vi "Data read test-Crossrulz.vi"() -> ()   [LabVIEW 2020]
uses:
  <vilib>/Instr/_visa.llb/VISA Configure Serial Port (Instr).vi
panel:
  out "Msg ID":string
  out "Header":string
  out "unsigned byte array":u8[](array[numeric])
  in  "Multicolumn Listbox":i32(listbox)
  out "error out":errorcluster
  in  "stop":bool
  in  "VISA resource name":refnum<visa-resource-name>
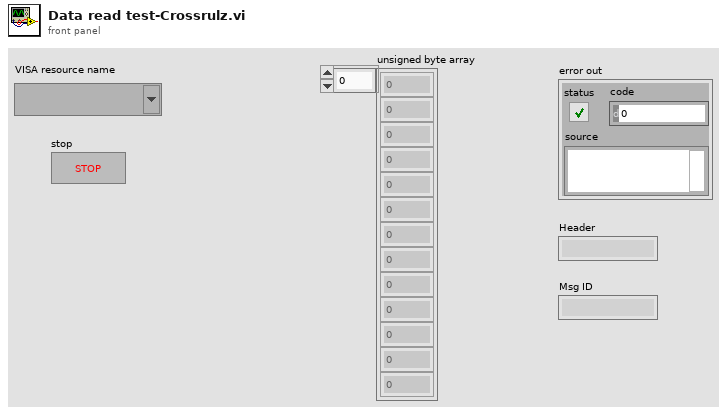
[diagram p1: front panel]
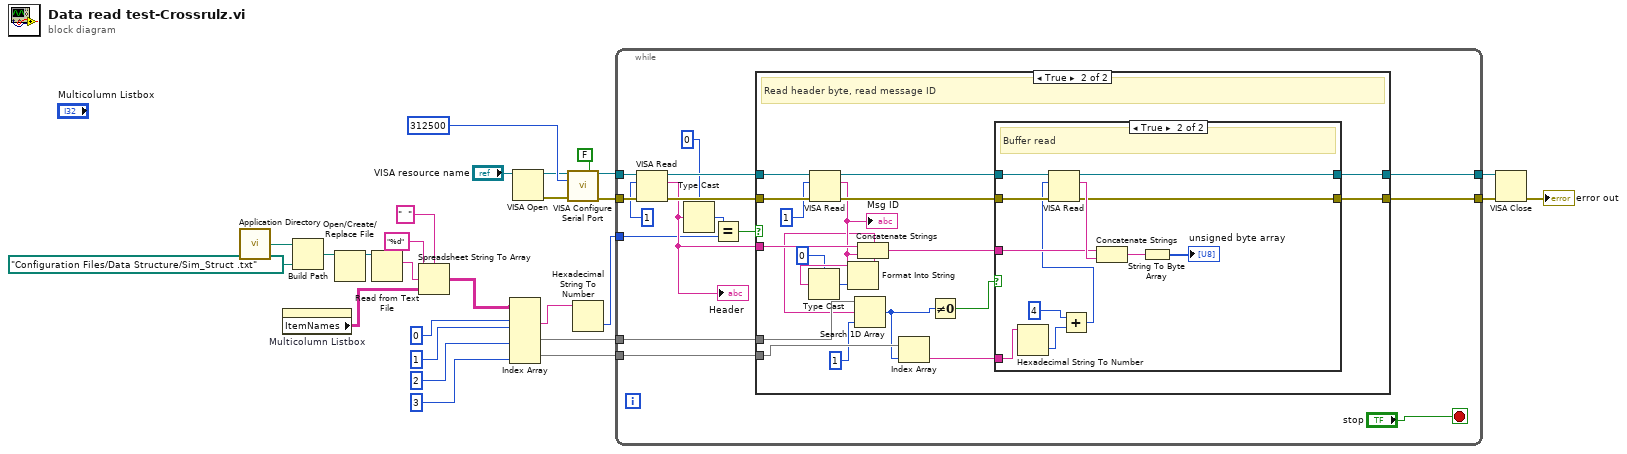
[diagram p0: block diagram]
diagram:
  n1 = call <vilib>:"Application Directory.vi"() -> ("Application Directory"=w16:path)
  n2 = property on="Multicolumn Listbox" class="MCListbox (strict)"() -> ("ItemNames"=w9:string[][])  [unwired: 2 in, 2 out]
  n3 = Build Path(base path=w16, name or relative path=path "Configuration Files/Data Structure/Sim_Struct .txt") -> (appended path=w14:path)
  n4 = Open/Create/Replace File(file path (use dialog)=w14) -> (refnum out=w13:refnum<file>)  [unwired: 5 in, 2 out]
  n5 = Read from Text File(file (use dialog)=w13) -> (text=w12:string)  [unwired: 3 in, 3 out]
  n6 = Spreadsheet String To Array(delimiter (Tab)="  ", format string="%d", spreadsheet string=w12, array type (2D Dbl)=w9) -> (array=w8:string[][])
  n7 = Index Array(array=w8, index (row) #1=0 ("index (row)"), index (col) #1=1 ("disabled index (col)"), index (col) #2=2 ("index (row)"), index (col) #3=3 ("index (col)")) -> (element #1=w2:string, element #2=w17:string[], element #3=w5:string[])  [unwired: 2 in]
  n8 = VISA Open(VISA resource name="VISA resource name") -> (VISA resource name=w4:refnum<visa-resource-name>, error out=w3:errorcluster)  [unwired: 4 in]
  n9 = call-poly "VISA Configure Serial Port"("VISA resource name"=w4, "Enable Termination\nChar (T)"=FALSE ("Enable Termination\nChar (T)"), "baud rate (9600)"=u32 312500, "error in (no error)"=w3) -> ("VISA resource name out"=w21:refnum<visa-resource-name>, "error out"=w27:errorcluster)  [unwired: 10 in]
  n10 = Hexadecimal String To Number(string=w2) -> (number=w1:u32)  [unwired: 2 in, 1 out]
  n11 = while {
    tunnel: w27 -> [w42]
    tunnel: w21 -> [w39]
    tunnel: [w35] -> w20
    tunnel: [w40] -> w26
    tunnel: w17 -> [w33]
    tunnel: w5 -> [w32]
    tunnel: w1 -> [w28]
    stop <- "stop" stop-if-true
    n12 = VISA Read(VISA resource name=w39, byte count=u32 1, error in (no error)=w42) -> (VISA resource name out=w37:refnum<visa-resource-name>, read buffer=w31:string, error out=w41:errorcluster)  [unwired: 1 out]
    "Header" <- w31
    n13 = Type Cast(type=u8 0, x=w31) -> (*(type *) &x=w29:u8)
    n14 = Equal?(x=w29, y=w28) -> (x = y?=w36:bool)
    n15 = case shown="True" w36 {
      tunnel: w37 -> [w43 w59]
      tunnel: w41 -> [w44 w63]
      tunnel: w31 -> [_ w57]
      tunnel: [w43 w55] -> w35
      tunnel: [w44 w61] -> w40
      tunnel: w33 -> [_ w54]
      tunnel: w32 -> [_ w53]
      frame False {
        # "Not the sync byte"
      }
      frame True {
        # "Read header byte, read message ID"
        n16 = VISA Read(VISA resource name=w59, byte count=u32 1, error in (no error)=w63) -> (VISA resource name out=w58:refnum<visa-resource-name>, read buffer=w48:string, error out=w62:errorcluster)  [unwired: 1 out]
        "Msg ID" <- w48
        n17 = Type Cast(type=u8 0, x=w48) -> (*(type *) &x=w46:u8)
        n18 = Format Into String(w46) -> (resulting string=w45:string)  [unwired: 3 in, 1 out]
        n19 = Search 1D Array(1D array=w54, element=w45, start index (0)=1) -> (index of element=w52:i32)
        n20 = Concatenate Strings(w57, w48) -> (w56:string)
        n21 = Index Array(array=w53, index=w52) -> (element=w50:string)
        n22 = Not Equal To 0?(x=w52) -> (x != 0?=w51:bool)
        n23 = case shown="True" w51 {
          tunnel: w58 -> [w64 w74]
          tunnel: w62 -> [w65 w76]
          tunnel: w56 -> [_ w73]
          tunnel: [w65 w75] -> w61
          tunnel: [w64 w71] -> w55
          tunnel: w50 -> [_ w70]
          frame False {
            # "Invalid ID.  Ignore."
          }
          frame True {
            # "Buffer read"
            n24 = Hexadecimal String To Number(string=w70) -> (number=w68:u32)  [unwired: 2 in, 1 out]
            n25 = Add(x=u32 4, y=w68) -> (x+y=w66:u32)
            n26 = VISA Read(VISA resource name=w74, byte count=w66, error in (no error)=w76) -> (VISA resource name out=w71:refnum<visa-resource-name>, read buffer=w77:string, error out=w75:errorcluster)  [unwired: 1 out]
            n27 = Concatenate Strings(w73, w77) -> (w72:string)
            n28 = String To Byte Array(string=w72) -> (unsigned byte array=→"unsigned byte array":u8[])
          }
        }
      }
    }
  }
  n29 = VISA Close(VISA resource name=w20, error in (no error)=w26) -> (error out=→"error out":errorcluster)
